vi "F Dwf Device Config Open.vi"(8 "error in (no error)":errorcluster, 9 "phdwf":i32, 10 "idxCfg":i32, 11 "idxDev":i32) -> (0 "error out":errorcluster, 1 "phdwf out":i32, 3 "function return":i32)   [LabVIEW 2021, in "Olasdwf.lvlib"]
doc: "DWFAPI int FDwfDeviceConfigOpen(int idxDev, int idxCfg, HDWF *phdwf);"
uses:
  Olasdwf.lvlib
  Windows/System32/dwf.dll
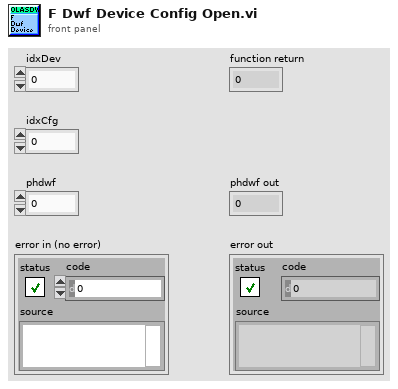
[diagram p1: front panel]
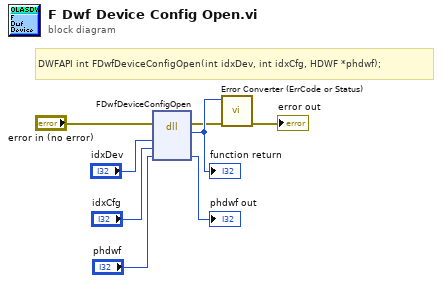
[diagram p0: block diagram]
diagram:
  # "DWFAPI int FDwfDeviceConfigOpen(int idxDev, int idxCfg, HDWF *phdwf);"
  n1 = dll-call lib="/Windows/System32/dwf.*" fn="FDwfDeviceConfigOpen"(error in="error in (no error)", "idxDev"="idxDev", "idxCfg"="idxCfg", "phdwf"="phdwf") -> (error out=w2:errorcluster, w8:i32, "phdwf"=→"phdwf out":i32)  [unwired: 4 in, 1 out]
  "function return" <- w8
  n2 = call "Error Converter (ErrCode or Status).vi"("error in (no error)"=w2, "error code"=w8) -> ("error out"=→"error out":errorcluster)  [unwired: 9 in]
